vi "Get HP5385A Data.vi"(8 "error in (no error)":errorcluster, 11 "VISA Resource Name":refnum<visa-resource-name>) -> (0 "error out":errorcluster, 1 "data":string, 2 "Frequency":dbl, 3 "VISA Resource Name Out":refnum<visa-resource-name>)   [LabVIEW 2015]
uses:
  GPIB/VISA  Send Receive.vi
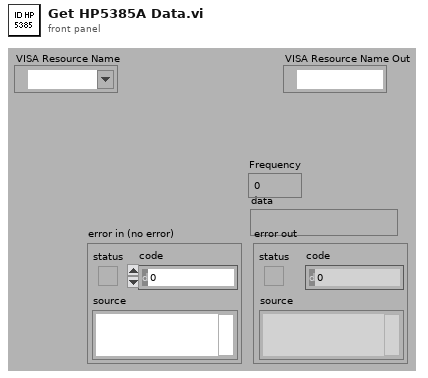
[diagram p1: front panel]
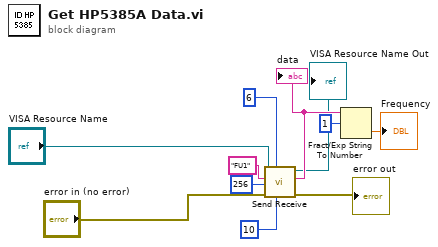
[diagram p0: block diagram]
diagram:
  n1 = call-poly "Send Receive.vi"("Read terminator"=i16 10, "Delay, ms"=u32 6, "error in (no error)"="error in (no error)", "Receive count"=256 ("byte count"), "data string in"="FU1", "VISA Resource Name"="VISA Resource Name") -> ("error out"=→"error out":errorcluster, "data string out"=w5:string, "VISA Resource Name Out"=→"VISA Resource Name Out":refnum<visa-resource-name>)  [unwired: 3 in]
  "data" <- w5
  n2 = Fract/Exp String To Number(string=w5, offset=1) -> (number=→"Frequency":dbl)  [unwired: 3 out]
